vi "UTC.vi"(8 "UTC":bool=TRUE, 11 "time stamp":timestamp) -> (0 "UTC format":bool=TRUE, 2 "Heure":string, 3 "Date":string)   [LabVIEW 2018]
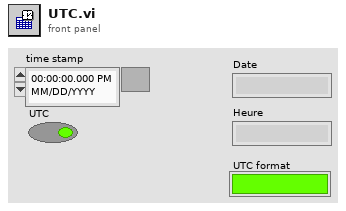
[diagram p1: front panel]
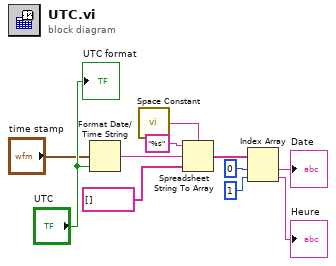
[diagram p0: block diagram]
diagram:
  n1 = Format Date/Time String(seconds (now)="time stamp", UTC format="UTC") -> (date/time string=w10:string)  [unwired: 1 in]
  n2 = call <vilib>:"Space Constant.vi"() -> ("String"=w7:string)
  n3 = Spreadsheet String To Array(delimiter (Tab)=w7, format string="%s", spreadsheet string=w10, array type (2D Dbl)=string[] []) -> (array=w6:string[])
  n4 = Index Array(array=w6, index #1=0 ("index"), index #2=1 ("index")) -> (element #1=→"Date":string, element #2=→"Heure":string)
  "UTC format" <- "UTC"
